vi "错误处理.vi"(8 "错误输入（无错误）":errorcluster, 11 "队列输入":refnum<queue>) -> (0 "错误输出":errorcluster)   [LabVIEW 2021]
uses:
  QueueLib/QueueLib.lvlib
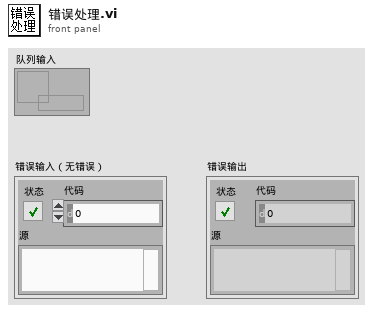
[diagram p1: front panel]
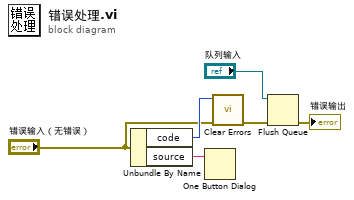
[diagram p0: block diagram]
diagram:
  n1 = Unbundle By Name("错误输入（无错误）") -> ("code"=w4:i32, "source"=w2:string)
  n2 = One Button Dialog(message=w2) -> ()  [unwired: 1 in, 1 out]
  n3 = call <vilib>:"Clear Errors.vi"("error in (no error)"="错误输入（无错误）", "specific error code to clear (0: all)"=w4) -> ("error out"=w3:errorcluster)  [unwired: 4 in, 1 out]
  n4 = Flush Queue(queue="队列输入", error in (no error)=w3) -> (error out=→"错误输出":errorcluster)  [unwired: 2 out]
